vi "fpga_check_range.vi"(6 "limit (low)":sgl, 7 "limit (high)":sgl, 11 "value":sgl) -> (3 "inrange?":bool)   [LabVIEW 2021]
doc: "This is sub vi for checking the threshold."
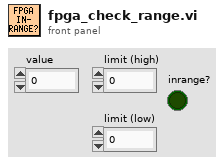
[diagram p1: front panel]
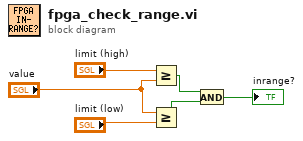
[diagram p0: block diagram]
diagram:
  n1 = Greater Or Equal?(x="limit (high)", y="value") -> (x >= y?=w1:bool)
  n2 = Greater Or Equal?(x="value", y="limit (low)") -> (x >= y?=w5:bool)
  n3 = And(x=w1, y=w5) -> (x .and. y?=→"inrange?":bool)
